vi "Connection_Arduino2.vi"(0 "VISA resource name":refnum<visa-resource-name>, 1 "baud rate (9600)":u32=115200) -> (2 "VISA resource name out":refnum<visa-resource-name>, 3 "error out":errorcluster, 4 "Arduino Conn":bool)   [LabVIEW 2018]
uses:
  <vilib>/Instr/_visa.llb/VISA Configure Serial Port (Instr).vi
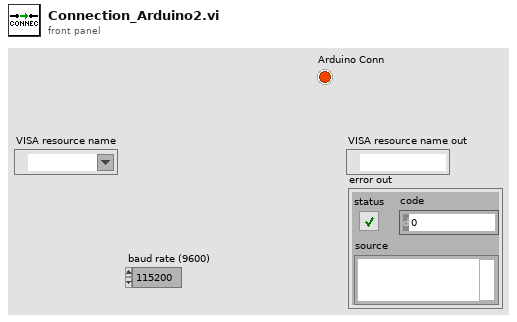
[diagram p1: front panel]
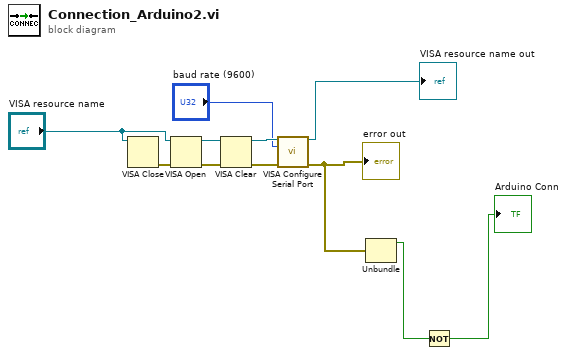
[diagram p0: block diagram]
diagram:
  n1 = VISA Close(VISA resource name="VISA resource name") -> (error out=w11:errorcluster)  [unwired: 1 in]
  n2 = VISA Open(error in (no error)=w11, VISA resource name="VISA resource name") -> (VISA resource name=w10:refnum<visa-resource-name>, error out=w9:errorcluster)  [unwired: 3 in]
  n3 = VISA Clear(VISA resource name=w10, error in (no error)=w9) -> (VISA resource name out=w7:refnum<visa-resource-name>, error out=w6:errorcluster)
  n4 = call-poly "VISA Configure Serial Port"("VISA resource name"=w7, "baud rate (9600)"="baud rate (9600)", "error in (no error)"=w6) -> ("VISA resource name out"=→"VISA resource name out":refnum<visa-resource-name>, "error out"=w3:errorcluster)  [unwired: 11 in]
  "error out" <- w3
  n5 = Unbundle(w3) -> ("status"=w1:bool)  [unwired: 2 out]
  n6 = Not(x=w1) -> (.not. x?=→"Arduino Conn":bool)
